vi "PAQmem_constructor.vi"(8 "error in (no error)":errorcluster, 9 "TAGs":string[](array[string]), 10 "LayerInfo":T1, 11 "PAQ-memory in":refnum<class "PAQ-memory.lvclass">) -> (0 "error out":errorcluster, 3 "PAQ-memory out":refnum<class "PAQ-memory.lvclass">)   [LabVIEW 2014, in "PAQ-memory.lvclass"]
uses:
  PAQ-memory.lvclass
  PAQ-memory.lvclass/PAQ-memory.ctl
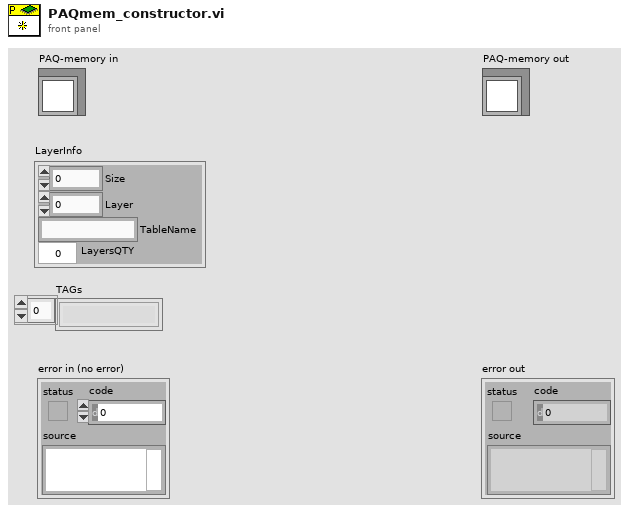
[diagram p1: front panel]
types:
  T1 = cluster{"Size":i32, "Layer":i32, "TableName":string, "LayersQTY":i32}
  T2 = cluster{"source":refnum<data-value>, "status":refnum<data-value>, "data":refnum<data-value>, "max":refnum<data-value>, "min":refnum<data-value>}
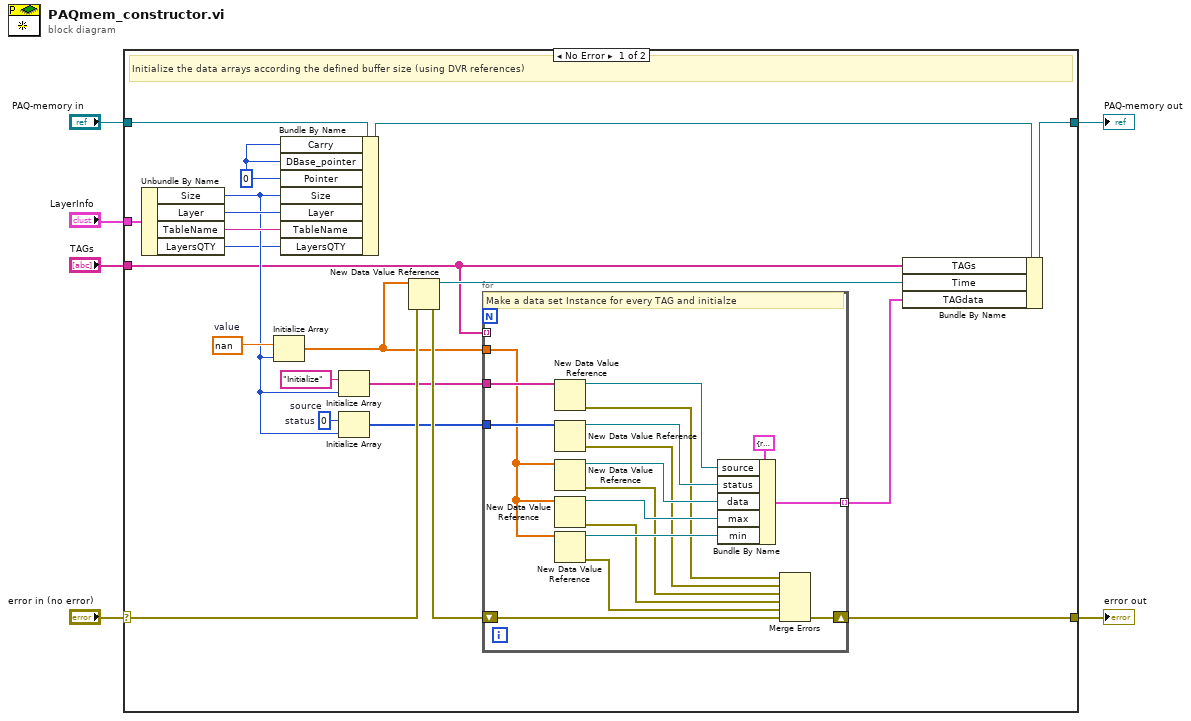
[diagram p0: block diagram]
diagram:
  n1 = case shown="No Error" "error in (no error)" {
    selector: "error in (no error)" -> [w17 w46]
    tunnel: [w14 w46] -> w1
    tunnel: [w18 w45] -> w2
    tunnel: "PAQ-memory in" -> [w24 w45]
    tunnel: "LayerInfo" -> [w27 _]
    tunnel: "TAGs" -> [w13 _]
    frame No Error {
      w20 = nan  # value
      w21 = u32 0  # status
      w22 = "Initialize"  # source
      w7 = 0 ("Pointer")
      # "Initialize the data arrays according the defined buffer size (using DVR references)"
      n2 = Unbundle By Name(w27) -> ("Size"=w16:i32, "Layer"=w26:i32, "TableName"=w25:string, "LayersQTY"=w12:i32)
      n3 = Initialize Array(w20, w16) -> (w11:dbl[])
      n4 = Bundle By Name(cluster=w24, "Carry"=w7, "DBase_pointer"=w7, "Pointer"=w7, "Size"=w16, "Layer"=w26, "TableName"=w25, "LayersQTY"=w12) -> (w23:refnum<class "PAQ-memory.lvclass">)
      n5 = Initialize Array(w22, w16) -> (w10:string[])
      n6 = Initialize Array(w21, w16) -> (w8:u32[])
      n7 = New Data Value Reference(data value=w11, error in=w17) -> (data value reference=w19:refnum<data-value>, error out=w15:errorcluster)
      n8 = for {
        tunnel: w11 -> [w37]
        tunnel: w10 -> [w39]
        shift-right: [w28] -> w14
        shift-left: w15 -> [w29]
        tunnel: w8 -> [w38]
        tunnel: [w35] -> w9 mode=indexing
        tunnel: w13 -> [_] mode=indexing
        # "Make a data set Instance for every TAG and initialze"
        n9 = New Data Value Reference(data value=w39) -> (data value reference=w44:refnum<data-value>, error out=w34:errorcluster)  [unwired: 1 in]
        n10 = New Data Value Reference(data value=w38) -> (data value reference=w43:refnum<data-value>, error out=w33:errorcluster)  [unwired: 1 in]
        n11 = New Data Value Reference(data value=w37) -> (data value reference=w42:refnum<data-value>, error out=w32:errorcluster)  [unwired: 1 in]
        n12 = New Data Value Reference(data value=w37) -> (data value reference=w41:refnum<data-value>, error out=w31:errorcluster)  [unwired: 1 in]
        n13 = New Data Value Reference(data value=w37) -> (data value reference=w40:refnum<data-value>, error out=w30:errorcluster)  [unwired: 1 in]
        n14 = Bundle By Name(cluster=T2 {"source"=refnum, "status"=refnum, "data"=refnum, "max"=refnum, "min"=refnum} ("TAGdata"), "source"=w44, "status"=w43, "data"=w42, "max"=w41, "min"=w40) -> (w35:T2)
        n15 = Merge Errors(w34, w33, w32, w31, w30, w29) -> (w28:errorcluster)
      }
      n16 = Bundle By Name(cluster=w23, "TAGs"=w13, "Time"=w19, "TAGdata"=w9) -> (w18:refnum<class "PAQ-memory.lvclass">)
    }
    frame Error {
      # "If error then empty all arrays"
    }
  }
  "error out" <- w1
  "PAQ-memory out" <- w2
